vi "2D Macro.vi"(5 "maximum":dbl, 6 "X,Y,Z Labels":string[](array[string])=["current (nA)", "field (oe)", "dV/dI (Ohm)"], 7 "minimum":dbl, 8 "error in (no error)":errorcluster, 10 "2D wavename":string="datatest.000016", 11 "ITX Commands in":refnum<class "ITX Commands.lvclass">) -> (0 "error out":errorcluster, 2 "Commands":string="Display;AppendImage 'datatest.000016'\nModifyGraph width=216,height={Aspect,1}\nLabel bottom \"current (nA)\"\nLabel left \"field (oe)\"\nModifyImage 'datatest.000016' ctab= {*,*,Rainbow,1}\n", 3 "ITX Commands out":refnum<class "ITX Commands.lvclass">)   [LabVIEW 2019, in "ITX Commands.lvclass"]
uses:
  ITX Commands.lvclass
  typedefs/Label--cluster.ctl
panel:
  # "Display;AppendImage '#wave2D#'\nModifyGraph width=216,height={Aspect,1}\nLabel bottom \"#labelX#\"\nLabel left \"#labelY#\"\nModifyImage '#wave2D#' ctab= {*,*,BlueHot,1}"
  # "Display;AppendImage '#wave2D#'\nModifyGraph width=216,height={Aspect,1}\nLabel bottom \"#labelX#\"\nLabel left \"#labelY#\"\nModifyImage '#wave2D#' ctab= {120,300,BlueHot,1}"
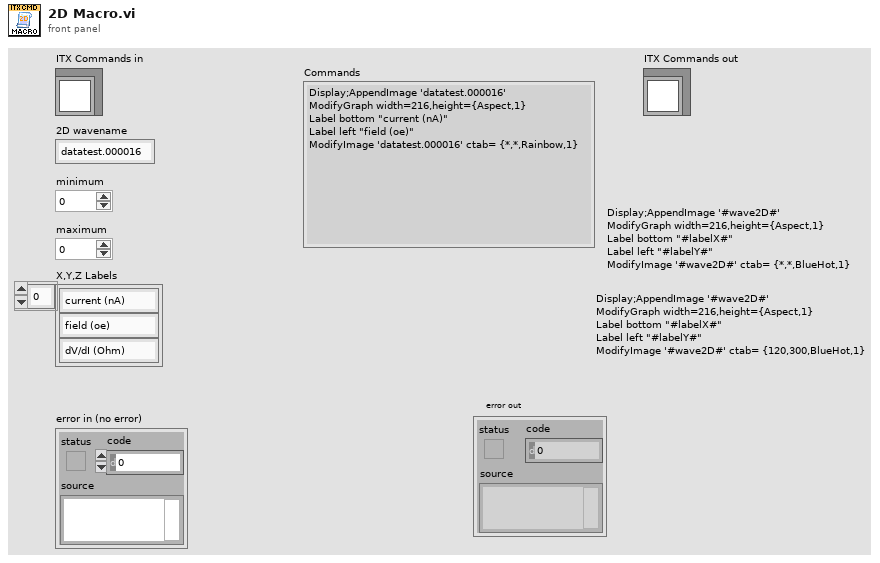
[diagram p1: front panel]
types:
  T1 = typedef "ITX Commands.lvclass/Label--cluster.ctl" = cluster{"Bottom":string, "Top":string, "Left":string, "Right":string}
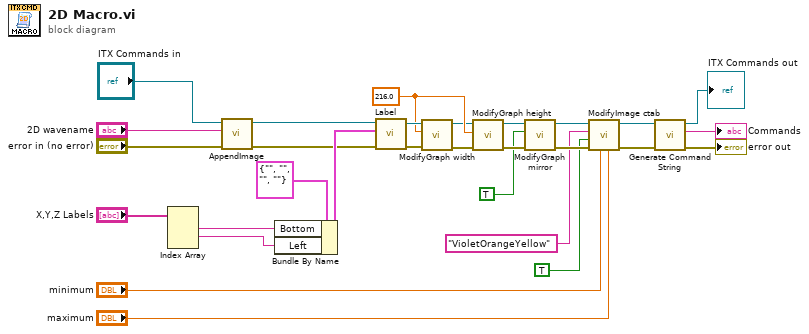
[diagram p0: block diagram]
diagram:
  w18 = 216.0 ("width (points) [256]")
  n1 = Index Array(array="X,Y,Z Labels") -> (element #1=w24:string, element #2=w23:string)  [unwired: 3 in, 1 out]
  n2 = call "AppendImage.vi"("error in (no error)"="error in (no error)", "wavename"="2D wavename", "ITX Commands in"="ITX Commands in") -> ("error out"=w22:errorcluster, "ITX Commands out"=w27:refnum<class "ITX Commands.lvclass">)  [unwired: 7 in]
  n3 = Bundle By Name(cluster=T1 {"Bottom"="", "Top"="", "Left"="", "Right"=""} ("Label"), "Bottom"=w24, "Left"=w23) -> (w25:T1)
  n4 = call "Label.vi"("error in (no error)"=w22, "Label"=w25, "ITX Commands in"=w27) -> ("error out"=w21:errorcluster, "ITX Commands out"=w20:refnum<class "ITX Commands.lvclass">)  [unwired: 7 in]
  n5 = call "ModifyGraph width.vi"("error in (no error)"=w21, "width (points) [256]"=w18, "ITX Commands in"=w20) -> ("error out"=w16:errorcluster, "ITX Commands out"=w17:refnum<class "ITX Commands.lvclass">)  [unwired: 7 in]
  n6 = call "ModifyGraph height.vi"("error in (no error)"=w16, "height (points) [256]"=w18, "ITX Commands in"=w17) -> ("error out"=w14:errorcluster, "ITX Commands out"=w15:refnum<class "ITX Commands.lvclass">)  [unwired: 7 in]
  n7 = call "ModifyGraph mirror.vi"("error in (no error)"=w14, "mirror [T]"=TRUE, "ITX Commands in"=w15) -> ("error out"=w9:errorcluster, "ITX Commands out"=w10:refnum<class "ITX Commands.lvclass">)  [unwired: 7 in]
  n8 = call "ModifyImage ctab.vi"("maximum"="maximum", "minimum"="minimum", "error in (no error)"=w9, "Invert Color Scheme? [NO]"=TRUE, "Color Table Name [VioletOrangeYellow]"="VioletOrangeYellow" ("Color Table Name [Rainbow]"), "ITX Commands in"=w10) -> ("error out"=w7:errorcluster, "ITX Commands out"=w8:refnum<class "ITX Commands.lvclass">)  [unwired: 4 in]
  n9 = call "Generate Command String.vi"("ITX Commands in"=w8, "error in (no error)"=w7) -> ("ITX Commands out"=→"ITX Commands out":refnum<class "ITX Commands.lvclass">, "ITX Commands"=→"Commands":string, "error out"=→"error out":errorcluster)  [unwired: 6 in]
